vi "notif_read.vi"(8 "error in (no error)":errorcluster) -> (0 "error out":errorcluster, 3 "latest notification":bool)   [LabVIEW 2020]
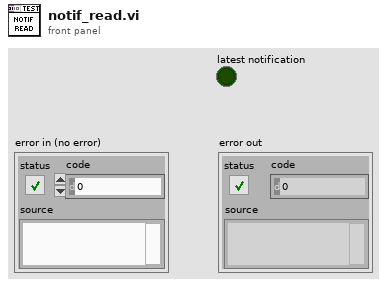
[diagram p1: front panel]
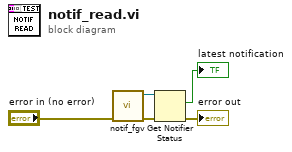
[diagram p0: block diagram]
diagram:
  n1 = call "notif_fgv.vi"("error in (no error)"="error in (no error)") -> ("error out"=w3:errorcluster, "notifier out"=w4:refnum<notifier>)  [unwired: 9 in]
  n2 = Get Notifier Status(notifier=w4, error in (no error)=w3) -> (current notification=→"latest notification":bool, error out=→"error out":errorcluster)  [unwired: 3 out]
